vi "pokretna traka.vi"() -> ()   [LabVIEW 2017]
uses:
  <vilib>/DAQmx/create/channels.llb/DAQmx Create Channel (DO-Digital Output).vi
  <vilib>/DAQmx/configure/timing.llb/DAQmx Timing (Sample Clock).vi
  <vilib>/DAQmx/create/channels.llb/DAQmx Create Channel (AI-Voltage-Basic).vi
  <vilib>/DAQmx/write.llb/DAQmx Write (Digital Bool 1Line 1Point).vi
  <vilib>/DAQmx/read.llb/DAQmx Read (Analog 1D DBL NChan 1Samp).vi
panel:
  out "odgovarajuca boja":bool
  out "gaudge":dbl(slide) scale=0.0..1000.0
  out "Image Out":T1(plugin-control)
  in  "PREDMET":enum16{"A", "B", "C"}(ring)
  in  "PROMENI PREDMET":bool
  in  "UKLONI ALARM":bool
  in  "POKRENI TRAKU":bool
  in  "PREDMET JE NA TRACI":bool
  in  "KRAJ RADA":bool
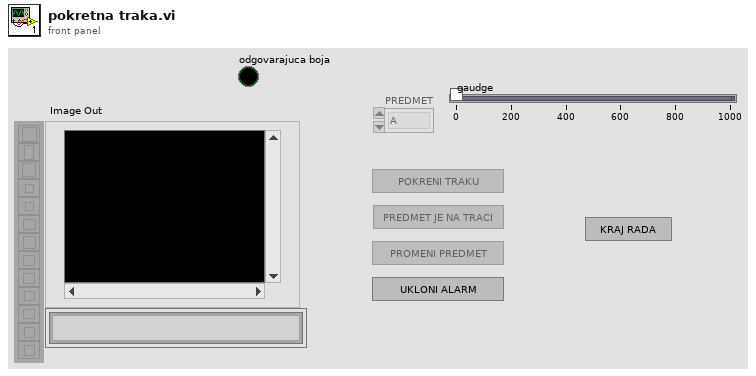
[diagram p1: front panel]
types:
  T1 = typedef "IMAQ Image.ctl" = refnum<image>
  T2 = enum16{"ALARM", "IZABERI", "CEKAJ", "MERENJE", "POKRENI", "SLIKANJE"}
  T3 = enum8{"Enabled", "Disabled", "Disabled and Grayed Out"}
  T4 = cluster{"MAX -masa":dbl, "MIN - masa":dbl, "PREDMET":enum16{"A", "B", "C"}}
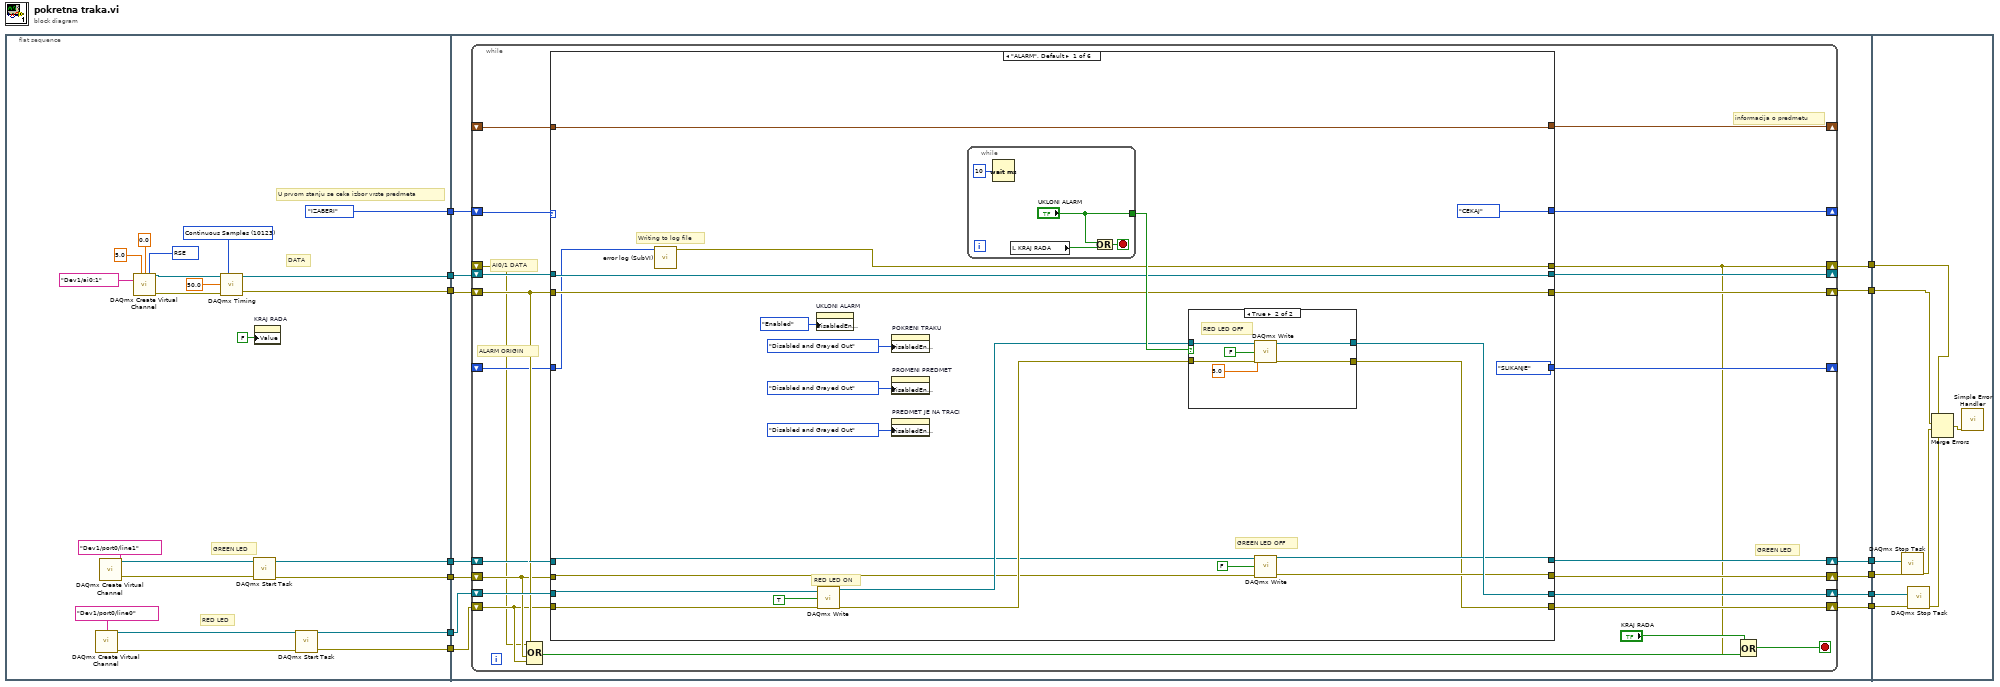
[diagram p0: block diagram]
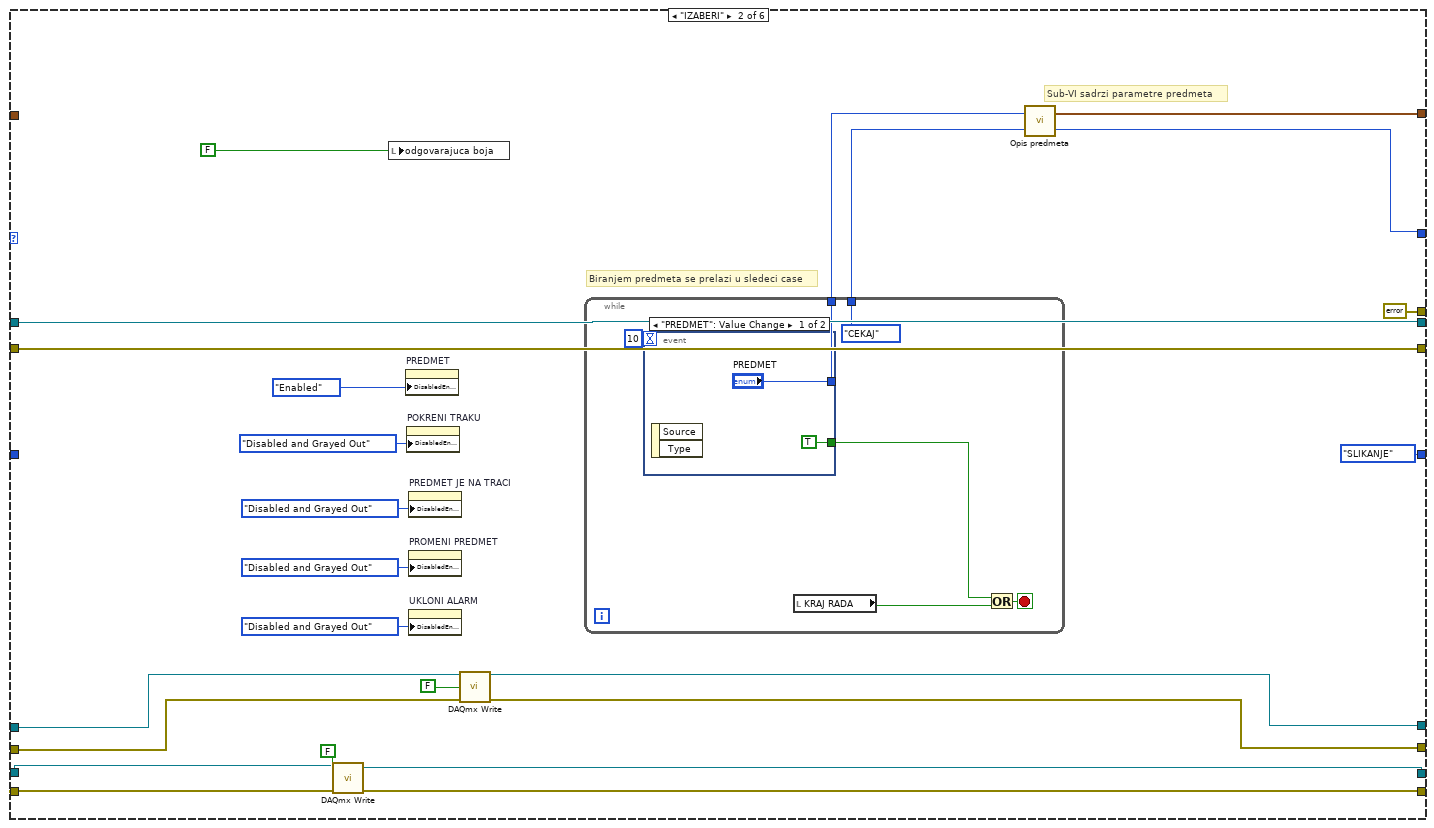
[diagram p3: hidden frame]
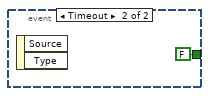
[diagram p4: hidden frame]
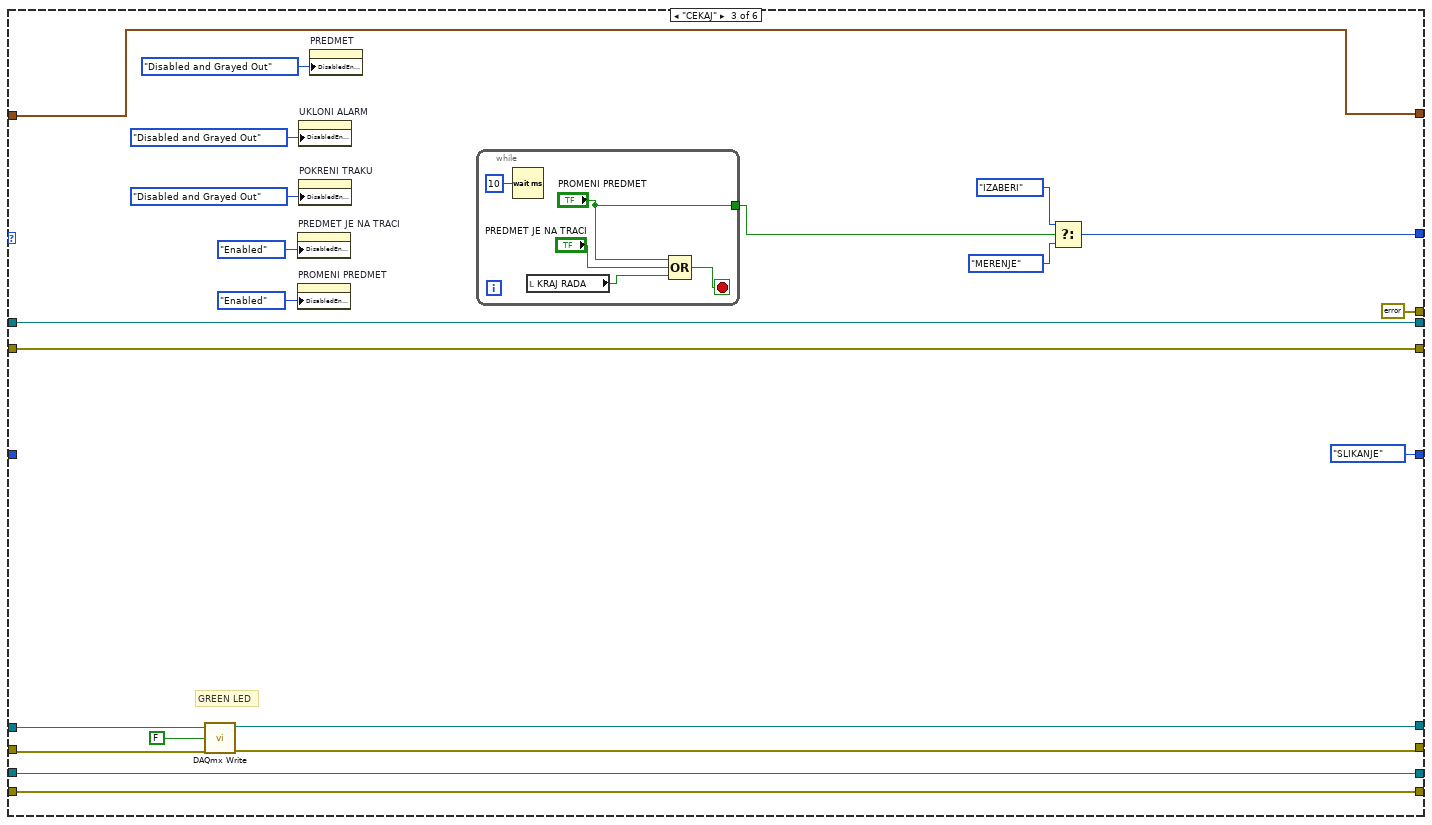
[diagram p5: hidden frame]
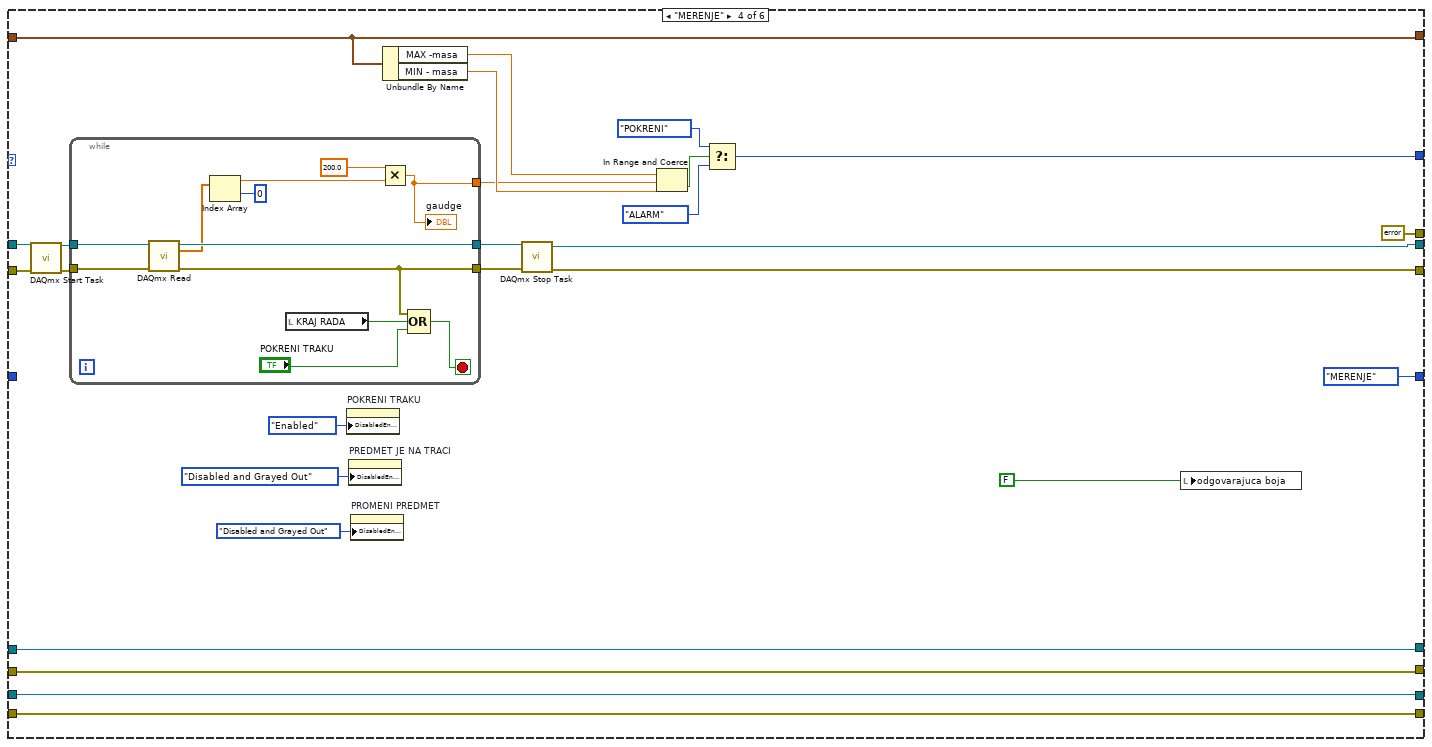
[diagram p6: hidden frame]
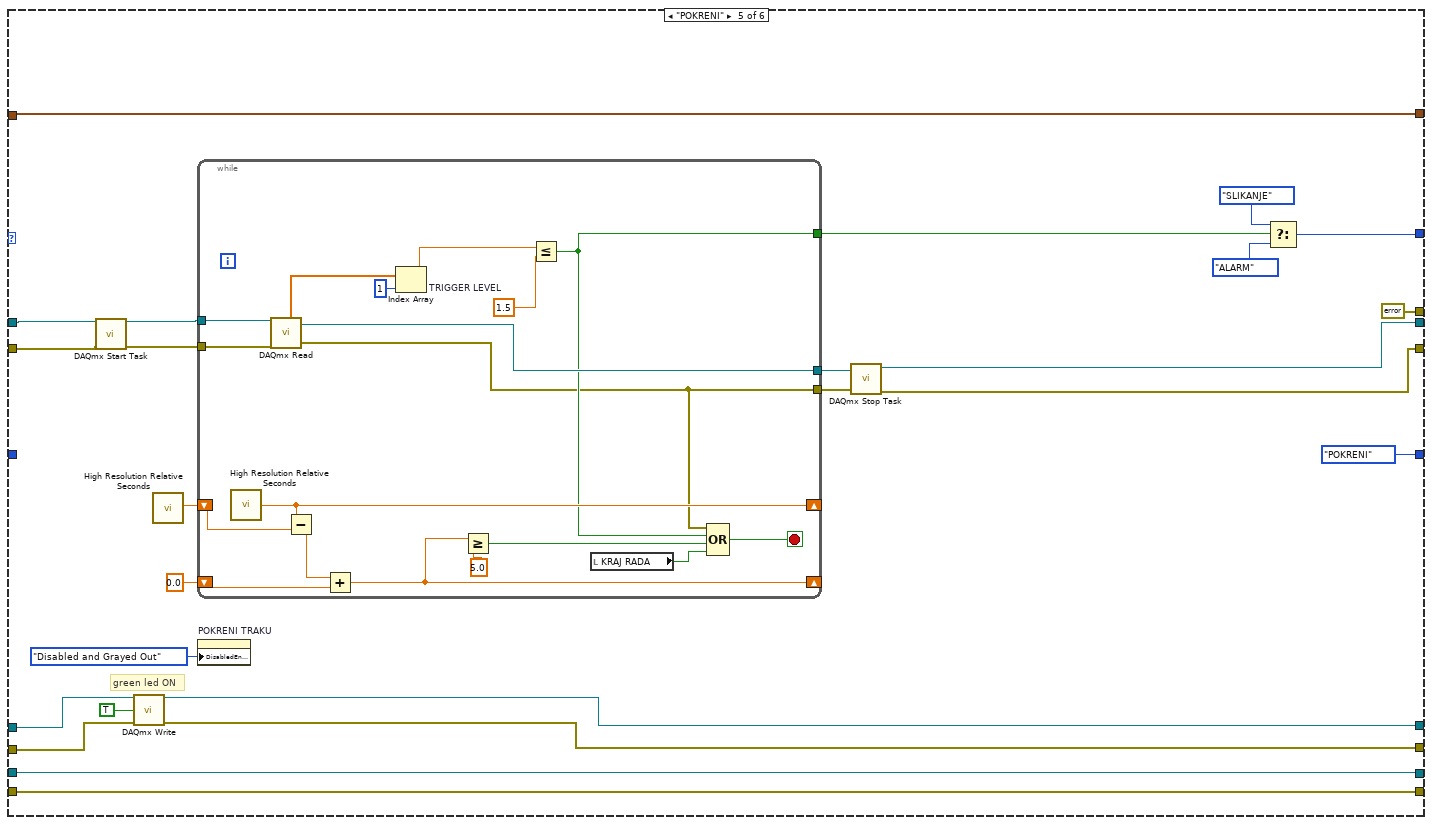
[diagram p7: hidden frame]
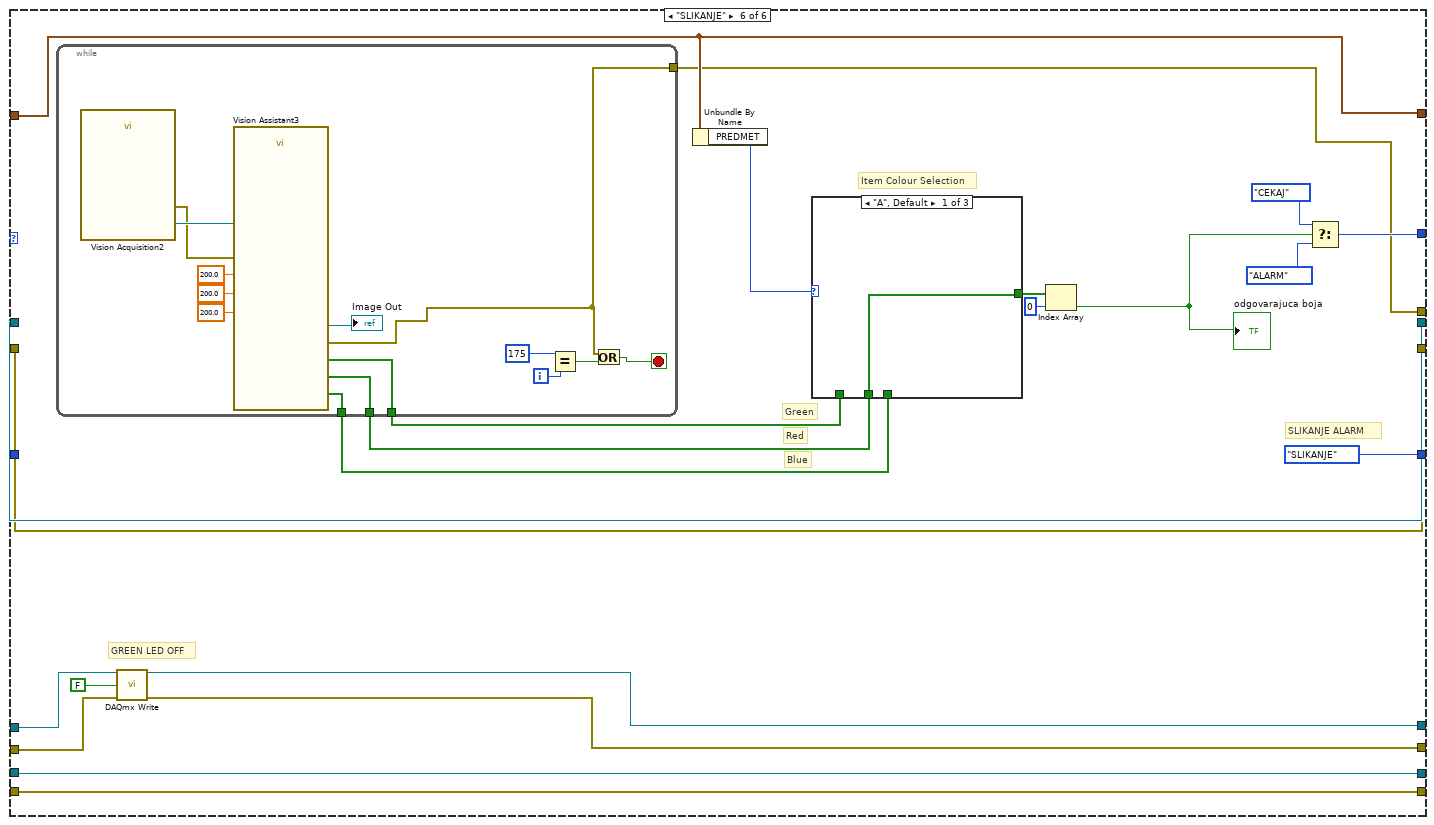
[diagram p8: hidden frame]
diagram:
  n1 = flat-sequence {
    tunnel: [T2."IZABERI"] -> w13
    tunnel: [w14] -> w12
    tunnel: [w15] -> w11
    tunnel: [w23] -> w9
    tunnel: [w22] -> w7
    tunnel: [w21] -> w6
    tunnel: [w20] -> w2
    tunnel: w13 -> [w48]
    tunnel: w12 -> [w43]
    tunnel: w11 -> [w44]
    tunnel: [w47] -> w10
    tunnel: w9 -> [w46]
    tunnel: [w39] -> w8
    tunnel: w7 -> [w37]
    tunnel: w6 -> [w38]
    tunnel: [w41] -> w5
    tunnel: [w42] -> w4
    tunnel: [w40] -> w3
    tunnel: w2 -> [w45]
    tunnel: [w36] -> w1
    tunnel: w10 -> [w287]
    tunnel: w8 -> [w295]
    tunnel: w5 -> [w294]
    tunnel: w4 -> [w293]
    tunnel: w3 -> [w292]
    tunnel: w1 -> [w288]
    frame #0 {
      w24 = 10123 items=["Finite Samples"=10178, "Continuous Samples"=10123, "Hardware Timed Single Point"=12522] ("sample mode")
      w28 = 10083 items=["Default"=-1, "RSE"=10083, "NRSE"=10078, "Differential"=10106, "Pseudodifferential"=12529] ("input terminal configuration")
      # "U prvom stanju se ceka izbor vrste predmeta"
      # "DATA"
      # "RED LED"
      # "GREEN LED"
      n2 = call-poly <vilib>:"DAQmx Create Virtual Channel.vi"("lines"=tag "Dev1/port0/line0") -> ("task out"=w32:refnum<k21>, "error out"=w31:errorcluster)  [unwired: 13 in]
      n3 = call-poly <vilib>:"DAQmx Create Virtual Channel.vi"("lines"=tag "Dev1/port0/line1") -> ("task out"=w34:refnum<k21>, "error out"=w33:errorcluster)  [unwired: 13 in]
      n4 = call-poly <vilib>:"DAQmx Create Virtual Channel.vi"("maximum value"=5.0, "minimum value"=0.0, "input terminal configuration"=w28, "physical channels"=tag "Dev1/ai0:1") -> ("task out"=w27:refnum<k21>, "error out"=w25:errorcluster)  [unwired: 10 in]
      n5 = call-poly <vilib>:"DAQmx Timing.vi"("task/channels in"=w27, "sample mode"=w24, "rate"=50.0, "error in"=w25) -> ("task out"=w15:refnum<k21>, "error out"=w14:errorcluster)  [unwired: 10 in]
      n6 = call <vilib>:"DAQmx Start Task.vi"("task/channels in"=w34, "error in"=w33) -> ("task out"=w23:refnum<k21>, "error out"=w20:errorcluster)  [unwired: 12 in]
      n7 = property on="KRAJ RADA" class="Bool (strict)"("Value"=FALSE ("KRAJ RADA")) -> ()  [unwired: 2 in, 2 out]
      n8 = call <vilib>:"DAQmx Start Task.vi"("task/channels in"=w32, "error in"=w31) -> ("task out"=w22:refnum<k21>, "error out"=w21:errorcluster)  [unwired: 12 in]
    }
    frame #1 {
      n9 = while {
        shift-right: [w70] -> _
        shift-left: w48 -> [w71]
        shift-right: [w69] -> _
        shift-left: _ -> [w68]
        shift-right: [w67] -> _
        shift-left: w44 -> [w61]
        shift-right: [w64] -> w47
        shift-left: w43 -> [w56]
        shift-right: [w58] -> w39
        shift-left: w46 -> [w66]
        shift-right: [w59] -> w40
        shift-left: w45 -> [w55]
        shift-right: [w60] -> w41
        shift-left: w37 -> [w65]
        shift-right: [w57] -> w42
        shift-left: w38 -> [w54]
        shift-right: [w52] -> _
        shift-left: _ -> [w51]
        shift-right: [w49] -> w36
        shift-left: _ -> [w50]
        stop <- w62 stop-if-true
        # "ALARM ORIGIN"
        # "AI0/1 DATA"
        # "GREEN LED"
        # "informacija o predmetu"
        n10 = Compound Arithmetic op=OR(w50, w56, w55, w54) -> (w53:bool)
        n11 = case shown="\"ALARM\", Default" w71 {
          tunnel: [T2."CEKAJ" w109 w156 w178 w224 w267] -> w70
          tunnel: [w95 w115 w145 w186 w228 w257] -> w69
          tunnel: w68 -> [w95 _ w145 w186 w228 w257]
          tunnel: w56 -> [w82 w125 w150 w173 w210 w268]
          tunnel: w61 -> [w83 w126 w151 w174 w211 w269]
          tunnel: [w83 w126 w151 w167 w207 w269] -> w67
          tunnel: [w82 w125 w150 w168 w206 w268] -> w64
          tunnel: w66 -> [w81 w124 w152 w183 w222 w263]
          tunnel: [w80 w113 w153 w183 w221 w258] -> w58
          tunnel: w65 -> [w88 w120 w149 w182 w220 w262]
          tunnel: w54 -> [w87 w119 w146 w180 w218 w261]
          tunnel: [w84 w118 w149 w182 w220 w262] -> w60
          tunnel: [w79 w114 w147 w181 w217 w259] -> w59
          tunnel: w55 -> [w78 w123 w148 w181 w216 w260]
          tunnel: [w76 w117 w146 w180 w218 w261] -> w57
          tunnel: [T2."SLIKANJE" T2."SLIKANJE" T2."SLIKANJE" T2."MERENJE" T2."POKRENI" T2."SLIKANJE"] -> w52
          tunnel: w51 -> [w73 _ _ _ _ _]
          tunnel: [w72 errorcluster {"status"=FALSE, "code"=0, "source"=""} ("error out") errorcluster {"status"=FALSE, "code"=0, "source"=""} ("error out") errorcluster {"status"=FALSE, "code"=0, "source"=""} ("error out") errorcluster {"status"=FALSE, "code"=0, "source"=""} ("error out") w249] -> w49
          frame "ALARM", Default {
            # "Writing to log file"
            # "GREEN LED OFF"
            # "RED LED ON"
            n12 = call "error log (SubVI).vi"("Enum"=w73) -> ("error out 2"=w72:errorcluster)  [unwired: 10 in]
            n13 = property on="UKLONI ALARM" class="Bool"("DisabledEnum"=T3."Enabled" ("Disabled")) -> ()  [unwired: 2 in, 2 out]
            n14 = call-poly <vilib>:"DAQmx Write.vi"("task/channels in"=w88, "data"=TRUE, "error in"=w87) -> ("task out"=w86:refnum<k21>, "error out"=w85:errorcluster)  [unwired: 10 in, 1 out]
            n15 = property on="POKRENI TRAKU" class="Bool"("DisabledEnum"=T3."Disabled and Grayed Out" ("Disabled")) -> ()  [unwired: 2 in, 2 out]
            n16 = property on="PROMENI PREDMET" class="Bool"("DisabledEnum"=T3."Disabled and Grayed Out" ("Disabled")) -> ()  [unwired: 2 in, 2 out]
            n17 = property on="PREDMET JE NA TRACI" class="Bool (strict)"("DisabledEnum"=T3."Disabled and Grayed Out" ("Disabled")) -> ()  [unwired: 2 in, 2 out]
            n18 = while {
              tunnel: ["UKLONI ALARM"] -> w90
              stop <- w98 stop-if-true
              n19 = Wait (ms)(milliseconds to wait=u32 10) -> ()  [unwired: 1 out]
              n20 = local read "KRAJ RADA"() -> (w97:bool)
              n21 = Or(x="UKLONI ALARM", y=w97) -> (x .or. y?=w98:bool)
            }
            n22 = case shown="True" w90 {
              tunnel: w86 -> [w101 w105]
              tunnel: w85 -> [w100 w104]
              tunnel: [w101 w103] -> w84
              tunnel: [w100 w102] -> w76
              frame False {
              }
              frame True {
                # "RED LED OFF"
                n23 = call-poly <vilib>:"DAQmx Write.vi"("task/channels in"=w105, "data"=FALSE, "timeout"=5.0, "error in"=w104) -> ("task out"=w103:refnum<k21>, "error out"=w102:errorcluster)  [unwired: 9 in, 1 out]
              }
            }
            n24 = call-poly <vilib>:"DAQmx Write.vi"("task/channels in"=w81, "data"=FALSE, "error in"=w78) -> ("task out"=w80:refnum<k21>, "error out"=w79:errorcluster)  [unwired: 10 in, 1 out]
          }
          frame "IZABERI" {
            # "Sub-VI sadrzi parametre predmeta"
            # "Biranjem predmeta se prelazi u sledeci case"
            n25 = call-poly <vilib>:"DAQmx Write.vi"("task/channels in"=w120, "data"=FALSE, "error in"=w119) -> ("task out"=w118:refnum<k21>, "error out"=w117:errorcluster)  [unwired: 10 in, 1 out]
            n26 = local write "odgovarajuca boja"(FALSE ("odgovarajuca boja")) -> ()
            n27 = property on="PREDMET" class="Enum (strict)"("DisabledEnum"=T3."Enabled" ("Disabled")) -> ()  [unwired: 2 in, 2 out]
            n28 = property on="POKRENI TRAKU" class="Bool"("DisabledEnum"=T3."Disabled and Grayed Out" ("Disabled")) -> ()  [unwired: 2 in, 2 out]
            n29 = property on="PREDMET JE NA TRACI" class="Bool (strict)"("DisabledEnum"=T3."Disabled and Grayed Out" ("Disabled")) -> ()  [unwired: 2 in, 2 out]
            n30 = property on="PROMENI PREDMET" class="Bool"("DisabledEnum"=T3."Disabled and Grayed Out" ("Disabled")) -> ()  [unwired: 2 in, 2 out]
            n31 = property on="UKLONI ALARM" class="Bool"("DisabledEnum"=T3."Disabled and Grayed Out" ("Disabled")) -> ()  [unwired: 2 in, 2 out]
            n32 = call-poly <vilib>:"DAQmx Write.vi"("task/channels in"=w124, "data"=FALSE, "error in"=w123) -> ("task out"=w113:refnum<k21>, "error out"=w114:errorcluster)  [unwired: 10 in, 1 out]
            n33 = while {
              tunnel: [T2."CEKAJ"] -> w110
              tunnel: [w132] -> w108
              stop <- w135 stop-if-true
              n34 = event shown="[0] \"PREDMET\": Value Change" {
                selector: _ -> [_ _]
                dyn-events: _ -> [_ _]
                timeout: 10 -> [_ _]
                tunnel: [TRUE FALSE] -> w134
                tunnel: ["PREDMET" _] -> w132
                event "PREDMET": Value Change {
                  n35 = event-data() -> ()  [unwired: 1 in, 2 out]
                }
                event Timeout {
                  n36 = event-data() -> ()  [unwired: 1 in, 2 out]
                }
              }
              n37 = local read "KRAJ RADA"() -> (w133:bool)
              n38 = Or(x=w134, y=w133) -> (x .or. y?=w135:bool)
            }
            n39 = call "Opis predmeta.vi"("Enum"=w110, "PREDMET"=w108) -> ("Enum 2"=w109:T2, "Opis predmeta"=w115:T4)
          }
          frame "CEKAJ" {
            # "GREEN LED"
            n40 = call-poly <vilib>:"DAQmx Write.vi"("task/channels in"=w152, "data"=FALSE, "error in"=w148) -> ("task out"=w153:refnum<k21>, "error out"=w147:errorcluster)  [unwired: 10 in, 1 out]
            n41 = property on="PREDMET JE NA TRACI" class="Bool (strict)"("DisabledEnum"=T3."Enabled" ("Disabled")) -> ()  [unwired: 2 in, 2 out]
            n42 = property on="PROMENI PREDMET" class="Bool"("DisabledEnum"=T3."Enabled" ("Disabled")) -> ()  [unwired: 2 in, 2 out]
            n43 = property on="UKLONI ALARM" class="Bool"("DisabledEnum"=T3."Disabled and Grayed Out" ("Disabled")) -> ()  [unwired: 2 in, 2 out]
            n44 = property on="POKRENI TRAKU" class="Bool"("DisabledEnum"=T3."Disabled and Grayed Out" ("Disabled")) -> ()  [unwired: 2 in, 2 out]
            n45 = property on="PREDMET" class="Enum (strict)"("DisabledEnum"=T3."Disabled and Grayed Out" ("Disabled")) -> ()  [unwired: 2 in, 2 out]
            n46 = while {
              tunnel: ["PROMENI PREDMET"] -> w141
              stop <- w163 stop-if-true
              n47 = Wait (ms)(milliseconds to wait=u32 10) -> ()  [unwired: 1 out]
              n48 = local read "KRAJ RADA"() -> (w165:bool)
              n49 = Compound Arithmetic op=OR("PROMENI PREDMET", "PREDMET JE NA TRACI", w165) -> (w163:bool)
            }
            n50 = Select(t=T2."IZABERI", s=w141, f=T2."MERENJE") -> (s? t:f=w156:T2)
          }
          frame "MERENJE" {
            n51 = call <vilib>:"DAQmx Start Task.vi"("task/channels in"=w174, "error in"=w173) -> ("task out"=w171:refnum<k21>, "error out"=w172:errorcluster)  [unwired: 12 in]
            n52 = while {
              tunnel: w172 -> [w204]
              tunnel: [w198] -> w169
              tunnel: w171 -> [w203]
              tunnel: [w202] -> w170
              tunnel: [w193] -> w177
              stop <- w199 stop-if-true
              n53 = call-poly <vilib>:"DAQmx Read.vi"("task/channels in"=w203, "error in"=w204) -> ("task out"=w202:refnum<k21>, "data"=w201:dbl[], "error out"=w198:errorcluster)  [unwired: 11 in]
              n54 = Index Array(array=w201, index=0 ("index (row)")) -> (element=w194:dbl)
              n55 = local read "KRAJ RADA"() -> (w197:bool)
              n56 = Multiply(x=200.0, y=w194) -> (x*y=w193:dbl)
              "gaudge" <- w193
              n57 = Compound Arithmetic op=OR(w198, w197, "POKRENI TRAKU") -> (w199:bool)
            }
            n58 = property on="POKRENI TRAKU" class="Bool"("DisabledEnum"=T3."Enabled" ("Disabled")) -> ()  [unwired: 2 in, 2 out]
            n59 = property on="PREDMET JE NA TRACI" class="Bool (strict)"("DisabledEnum"=T3."Disabled and Grayed Out" ("Disabled")) -> ()  [unwired: 2 in, 2 out]
            n60 = property on="PROMENI PREDMET" class="Bool"("DisabledEnum"=T3."Disabled and Grayed Out" ("Disabled")) -> ()  [unwired: 2 in, 2 out]
            n61 = Unbundle By Name(w186) -> ("MAX -masa"=w185:dbl, "MIN - masa"=w184:dbl)
            n62 = call <vilib>:"DAQmx Stop Task.vi"("task/channels in"=w170, "error in"=w169) -> ("task out"=w167:refnum<k21>, "error out"=w168:errorcluster)  [unwired: 12 in]
            n63 = In Range and Coerce(upper limit=w185, x=w177, lower limit=w184) -> (In Range?=w192:bool)  [unwired: 1 out]
            n64 = Select(t=T2."POKRENI", s=w192, f=T2."ALARM") -> (s? t:f=w178:T2)
            n65 = local write "odgovarajuca boja"(FALSE ("odgovarajuca boja")) -> ()
          }
          frame "POKRENI" {
            # "green led ON"
            n66 = call <vilib>:"DAQmx Start Task.vi"("task/channels in"=w211, "error in"=w210) -> ("task out"=w213:refnum<k21>, "error out"=w212:errorcluster)  [unwired: 12 in]
            n67 = call-poly <vilib>:"DAQmx Write.vi"("task/channels in"=w222, "data"=TRUE, "error in"=w216) -> ("task out"=w221:refnum<k21>, "error out"=w217:errorcluster)  [unwired: 10 in, 1 out]
            n68 = call <vilib>:"High Resolution Relative Seconds.vi"() -> ("relative seconds"=w205:dbl)
            n69 = while {
              tunnel: [w234] -> w227
              tunnel: [w230] -> w208
              tunnel: [w247] -> w209
              tunnel: w213 -> [w246]
              tunnel: w212 -> [w245]
              shift-right: [w242] -> _
              shift-left: w205 -> [w243]
              shift-right: [w239] -> _
              shift-left: 0.0 -> [w240]
              stop <- w231 stop-if-true
              w237 = 1.5  # TRIGGER LEVEL
              n70 = call <vilib>:"High Resolution Relative Seconds.vi"() -> ("relative seconds"=w242:dbl)
              n71 = call-poly <vilib>:"DAQmx Read.vi"("task/channels in"=w246, "error in"=w245) -> ("task out"=w247:refnum<k21>, "data"=w244:dbl[], "error out"=w230:errorcluster)  [unwired: 11 in]
              n72 = Subtract(x=w242, y=w243) -> (x-y=w241:dbl)
              n73 = Add(x=w241, y=w240) -> (x+y=w239:dbl)
              n74 = Index Array(array=w244, index=1) -> (element=w236:dbl)
              n75 = Greater Or Equal?(x=w239, y=5.0) -> (x >= y?=w233:bool)
              n76 = Less Or Equal?(x=w236, y=w237) -> (x <= y?=w234:bool)
              n77 = local read "KRAJ RADA"() -> (w232:bool)
              n78 = Compound Arithmetic op=OR(w230, w234, w233, w232) -> (w231:bool)
            }
            n79 = property on="POKRENI TRAKU" class="Bool"("DisabledEnum"=T3."Disabled and Grayed Out" ("Disabled")) -> ()  [unwired: 2 in, 2 out]
            n80 = call <vilib>:"DAQmx Stop Task.vi"("task/channels in"=w209, "error in"=w208) -> ("task out"=w207:refnum<k21>, "error out"=w206:errorcluster)  [unwired: 12 in]
            n81 = Select(t=T2."SLIKANJE", s=w227, f=T2."ALARM") -> (s? t:f=w224:T2)
          }
          frame "SLIKANJE" {
            # "SLIKANJE ALARM"
            # "Item Colour Selection"
            # "Blue"
            # "Red"
            # "Green"
            # "GREEN LED OFF"
            n82 = while {
              tunnel: [w282] -> w253
              tunnel: [w281] -> w254
              tunnel: [w280] -> w255
              tunnel: [w274] -> w249
              i -> [w273]
              stop <- w275 stop-if-true
              n83 = call "Vision Acquisition2"() -> ("Image Out"=w286:T1, "error out"=w283:errorcluster)  [unwired: 25 in, 1 out]
              n84 = call "Vision Assistant3"("Image In"=w286, "error in"=w283, "Minimum Match Score (GREEN)"=200.0, "Minimum Match Score (RED)"=200.0, "Minimum Match Score (BLUE)"=200.0) -> ("Image Out"=→"Image Out":T1, "error out"=w274:errorcluster, "Match Flag (GREEN)"=w280:bool[], "Match Flag (RED)"=w281:bool[], "Match Flag (BLUE)"=w282:bool[])  [unwired: 18 in]
              n85 = Equal?(x=u32 175 ("milliseconds to wait"), y=w273) -> (x = y?=w276:bool)
              n86 = Or(x=w274, y=w276) -> (x .or. y?=w275:bool)
            }
            n87 = call-poly <vilib>:"DAQmx Write.vi"("task/channels in"=w263, "data"=FALSE, "error in"=w260) -> ("task out"=w258:refnum<k21>, "error out"=w259:errorcluster)  [unwired: 10 in, 1 out]
            n88 = Unbundle By Name(w257) -> ("PREDMET"=w256:enum16{"A", "B", "C"})
            n89 = case shown="\"A\", Default" w256 {
              tunnel: w255 -> [_ w271 _]
              tunnel: w254 -> [w270 _ _]
              tunnel: w253 -> [_ _ w272]
              tunnel: [w270 w271 w272] -> w252
              frame "A", Default {
              }
              frame "B" {
              }
              frame "C" {
              }
            }
            n90 = Index Array(array=w252, index=0) -> (element=w251:bool)
            "odgovarajuca boja" <- w251
            n91 = Select(t=T2."CEKAJ", s=w251, f=T2."ALARM") -> (s? t:f=w267:T2)
          }
        }
        n92 = Compound Arithmetic op=OR("KRAJ RADA", w53, w49) -> (w62:bool)
      }
    }
    frame #2 {
      n93 = call <vilib>:"DAQmx Stop Task.vi"("task/channels in"=w295, "error in"=w292) -> ("error out"=w290:errorcluster)  [unwired: 12 in, 1 out]
      n94 = call <vilib>:"DAQmx Stop Task.vi"("task/channels in"=w294, "error in"=w293) -> ("error out"=w289:errorcluster)  [unwired: 12 in, 1 out]
      n95 = Merge Errors(w288, w287, w290, w289) -> (w291:errorcluster)
      n96 = call <vilib>:"Simple Error Handler.vi"("error in (no error)"=w291) -> ()  [unwired: 4 in, 5 out]
    }
  }
